vi "Init Config.vi"(8 "error in (no error)":errorcluster) -> (0 "error out":errorcluster)   [LabVIEW 2013]
uses:
  Data Access Objects/Metadata/LBCB Number.ctl
  Data Access Objects/Metadata/Persistant DAO Actions.ctl
  ConfigPathActions.ctl
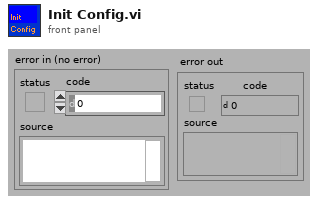
[diagram p1: front panel]
types:
  T1 = typedef "ConfigPathActions.ctl" = enum16{"Init", "Application", "MixedMode", "ControlLoop", "Calibration", "System", "Change Location"}
  T2 = typedef "Persistant DAO Actions.ctl" = enum16{"Init", "Get", "Set", "Load", "Save"}
  T3 = typedef "LBCB Number.ctl" = enum16{"LBCB1", "LBCB2"}
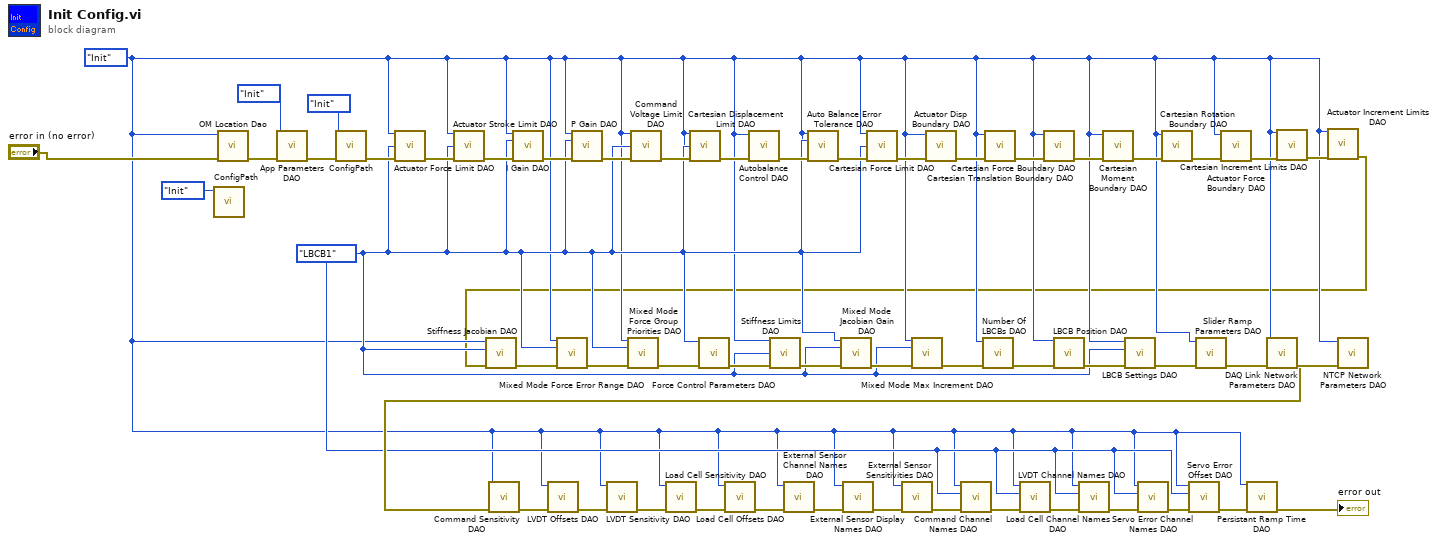
[diagram p0: block diagram]
diagram:
  w2 = Persistant_DAO_Actions."Init" ("Actions")
  w5 = LBCB_Number."LBCB1" ("LBCB Number")
  n1 = call "ConfigPath.vi"("Config Path Actions"=ConfigPathActions."Init") -> ()  [unwired: 2 in, 9 out]
  n2 = call "OM Location Dao.vi"("error in (no error)"="error in (no error)", "Actions"=w2) -> ("error out"=w30:errorcluster)  [unwired: 2 in, 7 out]
  n3 = call "App Parameters DAO.vi"("error in (no error)"=w30, "Actions"=Persistant_DAO_Actions."Init") -> ("error out"=w39:errorcluster)  [unwired: 2 in, 7 out]
  n4 = call "ConfigPath.vi"("error in (no error)"=w39, "Config Path Actions"=ConfigPathActions."Init") -> ("error out"=w38:errorcluster)  [unwired: 1 in, 8 out]
  n5 = call "Actuator Force Limit DAO.vi"("Actuator Force Limit Actions"=w2, "ID"=w5, "error in (no error)"=w38) -> ("error out"=w53:errorcluster)  [unwired: 2 in, 10 out]
  n6 = call "Actuator Stroke Limit DAO.vi"("Actuator Stroke Limit Actions"=w2, "ID"=w5, "error in (no error)"=w53) -> ("error out"=w52:errorcluster)  [unwired: 2 in, 10 out]
  n7 = call "I Gain DAO.vi"("I Gain Actions"=w2, "LBCB Number"=w5, "error in (no error)"=w52) -> ("error out"=w51:errorcluster)  [unwired: 2 in, 10 out]
  n8 = call "P Gain DAO.vi"("P Gain Actions"=w2, "LBCB Number"=w5, "error in (no error)"=w51) -> ("error out"=w50:errorcluster)  [unwired: 2 in, 10 out]
  n9 = call "Command Voltage Limit DAO.vi"("Actuator Stroke Limit Actions"=w2, "ID"=w5, "error in (no error)"=w50) -> ("error out"=w49:errorcluster)  [unwired: 2 in, 10 out]
  n10 = call "Cartesian Displacement Limit DAO.vi"("Cartesian Displacement Limit Actions"=w2, "ID"=w5, "error in (no error)"=w49) -> ("error out"=w48:errorcluster)  [unwired: 2 in, 10 out]
  n11 = call "Autobalance Control DAO.vi"("error in (no error)"=w48, "Persistent DAO Actions"=w2) -> ("error out"=w47:errorcluster)  [unwired: 2 in, 7 out]
  n12 = call "Auto Balance Error Tolerance DAO.vi"("Auto Balance Increment Actions"=w2, "LBCB Number"=w5, "error in (no error)"=w47) -> ("error out"=w46:errorcluster)  [unwired: 2 in, 10 out]
  n13 = call "Cartesian Force Limit DAO.vi"("Cartesian Force Limit Actions"=w2, "ID"=w5, "error in (no error)"=w46) -> ("error out"=w36:errorcluster)  [unwired: 2 in, 10 out]
  n14 = call "Actuator Disp Boundary DAO.vi"("error in (no error)"=w36, "Actions"=w2) -> ("error out"=w35:errorcluster)  [unwired: 2 in, 7 out]
  n15 = call "Cartesian Translation Boundary DAO.vi"("error in (no error)"=w35, "Actions"=w2) -> ("error out"=w34:errorcluster)  [unwired: 2 in, 7 out]
  n16 = call "Cartesian Force Boundary DAO.vi"("error in (no error)"=w34, "Actions"=w2) -> ("error out"=w33:errorcluster)  [unwired: 2 in, 7 out]
  n17 = call "Cartesian Moment Boundary DAO.vi"("error in (no error)"=w33, "Actions"=w2) -> ("error out"=w32:errorcluster)  [unwired: 2 in, 7 out]
  n18 = call "Cartesian Rotation Boundary DAO.vi"("error in (no error)"=w32, "Actions"=w2) -> ("error out"=w31:errorcluster)  [unwired: 2 in, 7 out]
  n19 = call "Actuator Force Boundary DAO.vi"("error in (no error)"=w31, "Actions"=w2) -> ("error out"=w4:errorcluster)  [unwired: 2 in, 7 out]
  n20 = call "Cartesian Increment Limits DAO.vi"("Actions"=w2, "error in (no error)"=w4) -> ("error out"=w3:errorcluster)  [unwired: 11 in, 2 out]
  n21 = call "Actuator Increment Limits DAO.vi"("Actions"=w2, "error in (no error)"=w3) -> ("error out"=w1:errorcluster)  [unwired: 11 in, 2 out]
  n22 = call "Stiffness Jacobian DAO.vi"("error in (no error)"=w1, "LBCB Number"=w5, "Actions"=w2) -> ("error out"=w45:errorcluster)  [unwired: 2 in, 6 out]
  n23 = call "Mixed Mode Force Error Range DAO.vi"("Force Error Range Actions"=w2, "LBCB Number"=w5, "error in (no error)"=w45) -> ("error out"=w9:errorcluster)  [unwired: 2 in, 10 out]
  n24 = call "Mixed Mode Force Group Priorities DAO.vi"("Force Error Range Actions"=w2, "LBCB Number"=w5, "error in (no error)"=w9) -> ("error out"=w8:errorcluster)  [unwired: 10 in, 2 out]
  n25 = call "Force Control Parameters DAO.vi"("error in (no error)"=w8, "DAO Actions"=w2) -> ("error out"=w7:errorcluster)  [unwired: 7 in, 2 out]
  n26 = call "Stiffness Limits DAO.vi"("Cartesian Force Limit Actions"=w2, "ID"=w5, "error in (no error)"=w7) -> ("error out"=w6:errorcluster)  [unwired: 10 in, 2 out]
  n27 = call "Mixed Mode Jacobian Gain DAO.vi"("Jacobian Gain Actions"=w2, "LBCB Number"=w5, "error in (no error)"=w6) -> ("error out"=w44:errorcluster)  [unwired: 2 in, 10 out]
  n28 = call "Mixed Mode Max Increment DAO.vi"("Max Increment Actions"=w2, "LBCB Number"=w5, "error in (no error)"=w44) -> ("error out"=w40:errorcluster)  [unwired: 2 in, 10 out]
  n29 = call "Number Of LBCBs DAO.vi"("error in (no error)"=w40, "Actions"=w2) -> ("error out"=w41:errorcluster)  [unwired: 3 in, 6 out]
  n30 = call "LBCB Position DAO.vi"("LBCB Settings Actions"=w2, "error in (no error)"=w41) -> ("error out"=w42:errorcluster)  [unwired: 3 in, 10 out]
  n31 = call "LBCB Settings DAO.vi"("error in (no error)"=w42, "LBCB Number"=w5, "Actions"=w2) -> ("error out"=w27:errorcluster)  [unwired: 2 in, 6 out]
  n32 = call "Slider Ramp Parameters DAO.vi"("error in (no error)"=w27, "Persistent DAO Actions"=w2) -> ("error out"=w12:errorcluster)  [unwired: 2 in, 7 out]
  n33 = call "DAQ Link Network Parameters DAO.vi"("error in (no error)"=w12, "Persistent DAO Actions"=w2) -> ("error out"=w11:errorcluster)  [unwired: 7 in, 2 out]
  n34 = call "NTCP Network Parameters DAO.vi"("error in (no error)"=w11, "Persistent DAO Actions"=w2) -> ("error out"=w10:errorcluster)  [unwired: 7 in, 2 out]
  n35 = call "Command Sensitivity DAO.vi"("error in (no error)"=w10, "Actions"=w2) -> ("error out"=w26:errorcluster)  [unwired: 3 in, 6 out]
  n36 = call "LVDT Offsets DAO.vi"("error in (no error)"=w26, "Actions"=w2) -> ("error out"=w25:errorcluster)  [unwired: 3 in, 6 out]
  n37 = call "LVDT Sensitivity DAO.vi"("error in (no error)"=w25, "Actions"=w2) -> ("error out"=w24:errorcluster)  [unwired: 3 in, 6 out]
  n38 = call "Load Cell Sensitivity DAO.vi"("error in (no error)"=w24, "Actions"=w2) -> ("error out"=w23:errorcluster)  [unwired: 3 in, 6 out]
  n39 = call "Load Cell Offsets DAO.vi"("error in (no error)"=w23, "Actions"=w2) -> ("error out"=w22:errorcluster)  [unwired: 3 in, 6 out]
  n40 = call "External Sensor Channel Names DAO.vi"("error in (no error)"=w22, "Persistent DAO Actions"=w2) -> ("error out"=w21:errorcluster)  [unwired: 2 in, 7 out]
  n41 = call "External Sensor Display Names DAO.vi"("error in (no error)"=w21, "Persistent DAO Actions"=w2) -> ("error out"=w20:errorcluster)  [unwired: 2 in, 7 out]
  n42 = call "External Sensor Sensitivities DAO.vi"("error in (no error)"=w20, "Persistent DAO Actions"=w2) -> ("error out"=w19:errorcluster)  [unwired: 2 in, 7 out]
  n43 = call "Command Channel Names DAO.vi"("error in (no error)"=w19, "LBCB Number"=w5, "Actions"=w2) -> ("error out"=w18:errorcluster)  [unwired: 2 in, 6 out]
  n44 = call "LVDT Channel Names DAO.vi"("error in (no error)"=w18, "LBCB Number"=w5, "Actions"=w2) -> ("error out"=w17:errorcluster)  [unwired: 2 in, 6 out]
  n45 = call "Load Cell Channel Names DAO.vi"("error in (no error)"=w17, "LBCB Number"=w5, "Actions"=w2) -> ("error out"=w16:errorcluster)  [unwired: 2 in, 6 out]
  n46 = call "Servo Error Channel Names DAO.vi"("error in (no error)"=w16, "LBCB Number"=w5, "Actions"=w2) -> ("error out"=w15:errorcluster)  [unwired: 2 in, 6 out]
  n47 = call "Servo Error Offset DAO.vi"("error in (no error)"=w15, "LBCB Number"=w5, "Actions"=w2) -> ("error out"=w14:errorcluster)  [unwired: 2 in, 6 out]
  n48 = call "Persistant Ramp Time DAO.vi"("Ramp Time Actions"=w2, "error in (no error)"=w14) -> ("error out"=→"error out":errorcluster)  [unwired: 2 in, 11 out]
